vi "Position Altitude Slider.vi"(8 "error in (no error)":errorcluster, 10 "Previous Button":refnum<vi>, 11 "Num Refnum":refnum<vi>) -> (0 "error out":errorcluster)   [LabVIEW 2014]
panel:
  in  "Desired Altitude (m)":dbl=20.0 step=1.0
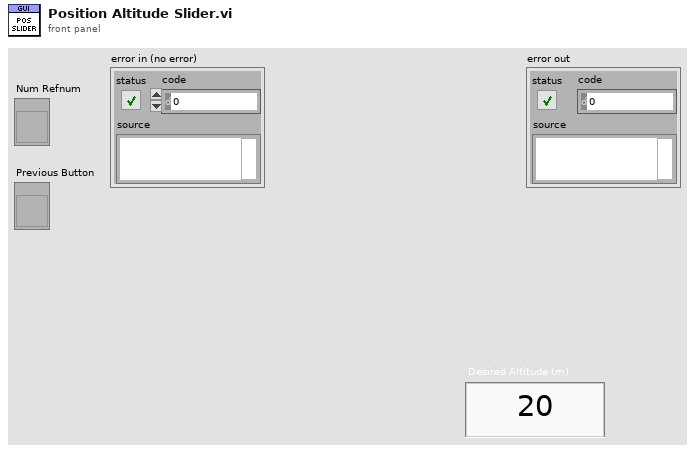
[diagram p1: front panel]
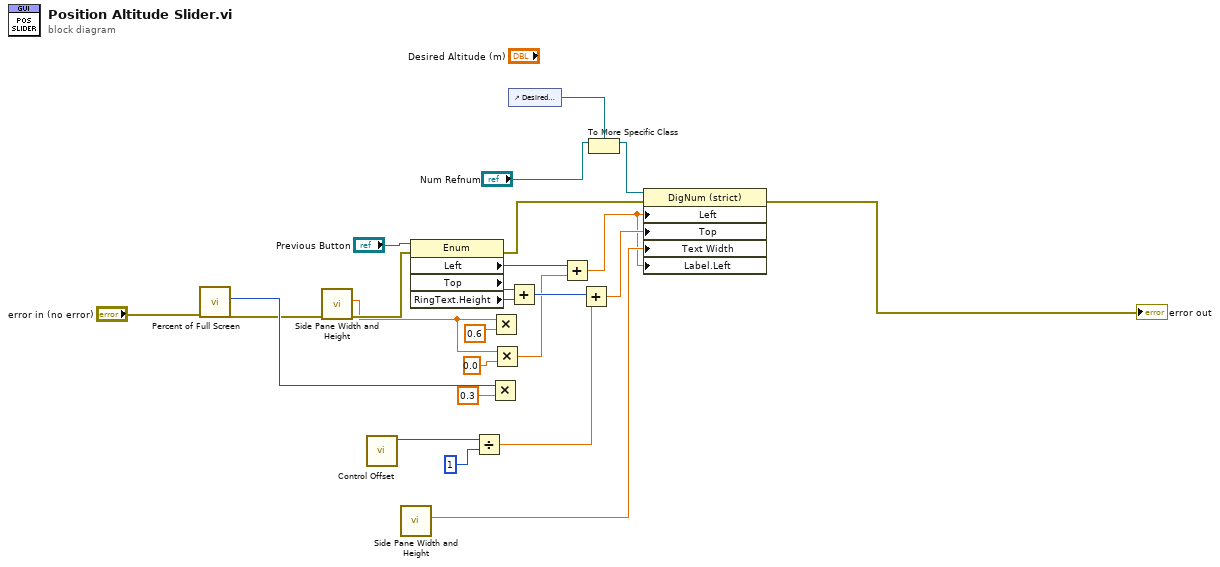
[diagram p0: block diagram]
diagram:
  n1 = call "Percent of Full Screen.vi"("error in (no error)"="error in (no error)") -> ("error out"=w11:errorcluster, "Bottom"=w21:i16)  [unwired: 8 in, 1 out]
  n2 = call "Side Pane Width and Height.vi"("error in (no error)"=w11) -> ("error out"=w12:errorcluster, "Width"=w9:dbl)  [unwired: 8 in, 1 out]
  n3 = call "Control Offset.vi"() -> ("Offset From Tab Edge in (px)"=w16:i32)  [unwired: 11 in]
  n4 = call "Side Pane Width and Height.vi"() -> ("Width"=w2:dbl)  [unwired: 9 in, 2 out]
  n5 = property class="Enum"(reference="Previous Button", error in=w12) -> (error out=w19:errorcluster, "Left"=w10:i32, "Top"=w24:i32, "RingText.Height"=w23:u32)  [unwired: 1 out]
  n6 = Divide(x=w16, y=1) -> (x/y=w13:dbl)
  n7 = Multiply(x=w21, y=0.3) -> ()  [unwired: 1 out]
  n8 = Multiply(x=w9, y=0.6) -> ()  [unwired: 1 out]
  n9 = Multiply(x=w9, y=0.0) -> (x*y=w7:dbl)
  n10 = control-ref of="Desired Altitude (m)"() -> (w5:refnum<vi>)
  n11 = Add(x=w24, y=w23) -> (x+y=w18:u32)
  n12 = Add(x=w10, y=w7) -> (x+y=w1:dbl)
  n13 = Add(x=w18, y=w13) -> (x+y=w14:dbl)
  n14 = To More Specific Class(target class=w5, reference="Num Refnum") -> (specific class reference=w4:refnum<vi>)  [unwired: 1 in, 1 out]
  n15 = property class="DigNum (strict)"(reference=w4, error in=w19, "Left"=w1, "Top"=w14, "Text Width"=w2, "Label.Left"=w1) -> (error out=→"error out":errorcluster)  [unwired: 1 out]
